vi "FT10_Fornax Command.vi"(11 "ExternalCommCommand":T1(ring)) -> (3 "JSON Message":string)   [LabVIEW 2015]
doc: "Converts enum command into JSON string that can be written to Fornax via TCP.\n\nCopy of \"Fornax_Write_ExternalCommCommand.vi\" from \"HWT_Power Curve Test.lvproj\""
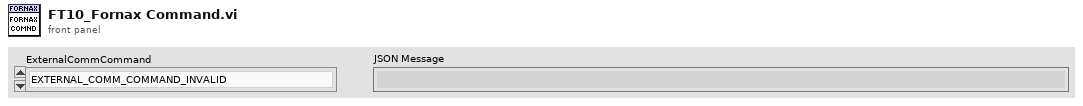
[diagram p1: front panel]
types:
  T1 = enum16{"EXTERNAL_COMM_COMMAND_INVALID", "EXTERNAL_COMM_COMMAND_PAIR_VLEX", "EXTERNAL_COMM_COMMAND_PAIR_FORNAX", "EXTERNAL_COMM_COMMAND_PAIR_INTEGRATION_TESTOR", "EXTERNAL_COMM_COMMAND_ENABLE_DFA", "EXTERNAL_COMM_COMMAND_ENABLE_DFT", "EXTERNAL_COMM_COMMAND_ENABLE_VIPER", "EXTERNAL_COMM_COMMAND_AUTO_ETHERNET_ON", "EXTERNAL_COMM_COMMAND_AUTO_ETHERNET_OFF", "EXTERNAL_COMM_COMMAND_STREAM_RFDATA_ON", "EXTERNAL_COMM_COMMAND_STREAM_RFDATA_OFF", "EXTERNAL_COMM_COMMAND_STREAM_ISOFIRM_ON", "EXTERNAL_COMM_COMMAND_STREAM_ISOFIRM_OFF", "EXTERNAL_COMM_COMMAND_STREAM_RFID_ON", "EXTERNAL_COMM_COMMAND_STREAM_RFID_OFF", "EXTERNAL_COMM_COMMAND_AUTO_ETHERNET_ONCE"}
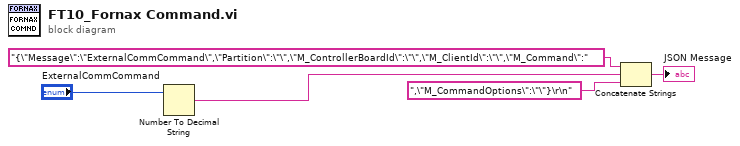
[diagram p0: block diagram]
diagram:
  n1 = Number To Decimal String(number="ExternalCommCommand") -> (decimal integer string=w3:string)  [unwired: 1 in]
  n2 = Concatenate Strings("{\"Message\":\"ExternalCommCommand\",\"Partition\":\"\",\"M_ControllerBoardId\":\"\",\"M_ClientId\":\"\",\"M_Command\":", w3, ",\"M_CommandOptions\":\"\"}\r\n") -> (→"JSON Message":string)
